vi "MetaWaitServer.vi"   [LabVIEW 2017]
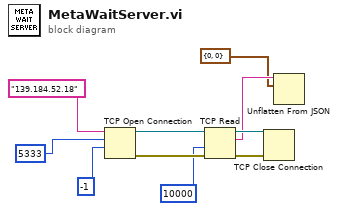
[diagram p0: block diagram]
diagram:
  n1 = TCP Open Connection(address="139.184.52.18", remote port or service name=u16 5333, timeout ms (60000)=-1) -> (connection ID=w10:refnum<k5>, error out=w9:errorcluster)  [unwired: 2 in]
  n2 = TCP Read(connection ID=w10, error in (no error)=w9, 9:10000 ("timeout ms (25000)")) -> (connection ID out=w6:refnum<k5>, data out=w5:string, error out=w7:errorcluster)  [unwired: 2 in]
  n3 = TCP Close Connection(connection ID=w6, error in (no error)=w7) -> ()  [unwired: 1 in, 2 out]
  n4 = Unflatten From JSON(JSON string=w5, type and defaults=cluster{"steps":i32, "runs":i32} {"steps"=0, "runs"=0}) -> ()  [unwired: 5 in, 2 out]
